vi "Autonomous Independent.vi"() -> ()   [LabVIEW 2012]
doc: "This VI is called when autonomous begins, and will automatically be terminated when autonomous ends. You can carry out timed or sensor driven robot movement independently without needing to return to the caller."
uses:
  <vilib>/Rock Robotics/WPI/Relay/WPI_RelayValue.ctl
  Robot Global Data.vi
  <vilib>/Rock Robotics/WPI/RobotDrive/WPI_RobotDriveGetSetRefNum.vi
  <vilib>/Rock Robotics/WPI/RobotDrive/WPI_RobotDriveArcadeDrive_Standard(NoSaturation).vi
panel:
  out "Current Movement, for debugging":T1 {"Y Joystick Value" scale=1.0..-1.0; "X Joystick Value" scale=-1.0..1.0}
  in  "Array of robot movements":T2(array[cluster]) {"Y Joystick Value" scale=1.0..-1.0; "X Joystick Value" scale=-1.0..1.0}
  # "Be sure to right-click and choose Data Operations>>Make Current Value default if you want to save the array values with the VI"
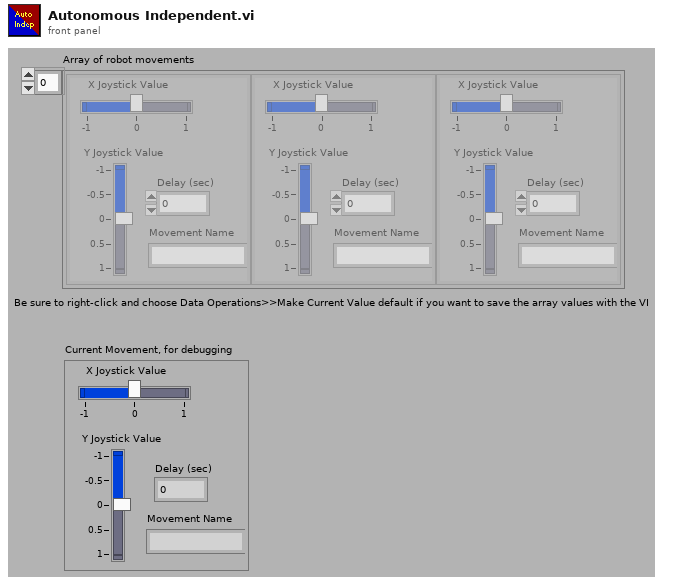
[diagram p1: front panel]
types:
  T1 = cluster{"X Joystick Value":dbl, "Y Joystick Value":dbl, "Delay (sec)":dbl, "Movement Name":string}
  T2 = cluster{"X Joystick Value":dbl, "Y Joystick Value":dbl, "Delay (sec)":dbl, "Movement Name":string}[]
  T3 = typedef "WPI_JoystickDevRef.ctl" = cluster{"Device":T4}
  T4 = typedef "WPI_JoystickDeviceEnum.ctl" = enum16{"USB 1", "USB 2", "USB 3", "USB 4", "Kinect 1", "Kinect 2"}
  T5 = cluster{"axis 1 (x)":dbl, "axis 2 (y)":dbl, "axis 3 (throttle)":dbl, "axis 4":dbl, "axis 5":dbl, "axis 6":dbl}
  T6 = typedef "WPI_RobotDriveDevRef.ctl" = cluster{"DevStatus":errorcluster, "Motors[]":T7[], "Square Inputs":bool, "Max Output":dbl, "Isochronous":bool}
  T7 = typedef "WPI_MotorControlDeviceRef.ctl" = cluster{"DeviceStatus":errorcluster, "Type":enum16{"PWM", "CAN"}, "PWM":cluster{"Digital Module":T8, "PWM Channel":T9, "DeadBand":T10}, "CAN":cluster{"Device Number":u8, "Control Mode":T11, "Semaphore":T12, "Max Vout":dbl}, "Invert":bool, "TransformRef":T13, "InvTransformRef":T13}
  T8 = typedef "FPGA_TypedefDigitalModule.ctl" = enum16{"Digital Module 1", "Digital Module 2"}
  T9 = typedef "FPGA_DIOPWMChannel.ctl" = enum8{"PWM 1", "PWM 2", "PWM 3", "PWM 4", "PWM 5", "PWM 6", "PWM 7", "PWM 8", "PWM 9", "PWM 10", "Invalid"}
  T10 = typedef "WPI_PWMDeadband.ctl" = cluster{"Name":string, "maxPositivePwm":i32, "minPositivePwm":i32, "centerPwm":i32, "maxNegativePwm":i32, "minNegativePwm":i32, "angularRange":u16}
  T11 = typedef "WPI_CANJaguar_ControlMode.ctl" = enum8{"Percent VBus", "Current", "Speed", "Position", "Voltage"}
  T12 = typedef "Semaphore RefNum" = refnum<k1>
  T13 = typedef "WPI_PWMTransform_ConPane.ctl" = refnum<vi>
  T14 = typedef "WPI_RelayValue.ctl" = enum16{"Off", "On", "Forward", "Reverse"}
  T15 = typedef "WPI_RelayDevRef.ctl" = cluster{"DevStatus":errorcluster, "Relay Channel":T16, "Digital Module":T8, "Relay Direction":T17}
  T16 = typedef "FPGA_DIORelayChannel.ctl" = enum8{"Relay 1", "Relay 2", "Relay 3", "Relay 4", "Relay 5", "Relay 6", "Relay 7", "Relay 8", "Invalid"}
  T17 = typedef "WPI_RelayDirection.ctl" = enum16{"Both directions", "Forward only", "Reverse only"}
  T18 = typedef "WPI_EncoderDevRef.ctl" = cluster{"DevStatus":errorcluster, "EncoderIndex":T19, "CounterIndex":T20, "DistancePerCount":dbl, "Decoding Type":T21}
  T19 = typedef "FPGA_EncoderIdx.ctl" = enum8{"Enc 0", "Enc 1", "Enc 2", "Enc 3", "Invalid"}
  T20 = typedef "FPGA_CounterCtrSystemIndex.ctl" = enum8{"Ctr 0", "Ctr 1", "Ctr 2", "Ctr 3", "Ctr 4", "Ctr 5", "Ctr 6", "Ctr 7", "Invalid"}
  T21 = typedef "WPI_EncoderType.ctl" = enum16{"1x", "2x", "4x"}
  T22 = typedef "WPI_ServoDeviceRef.ctl" = cluster{"DeviceStatus":errorcluster, "Digital Module":T8, "PWM Channel":T9, "DeadBand":T10}
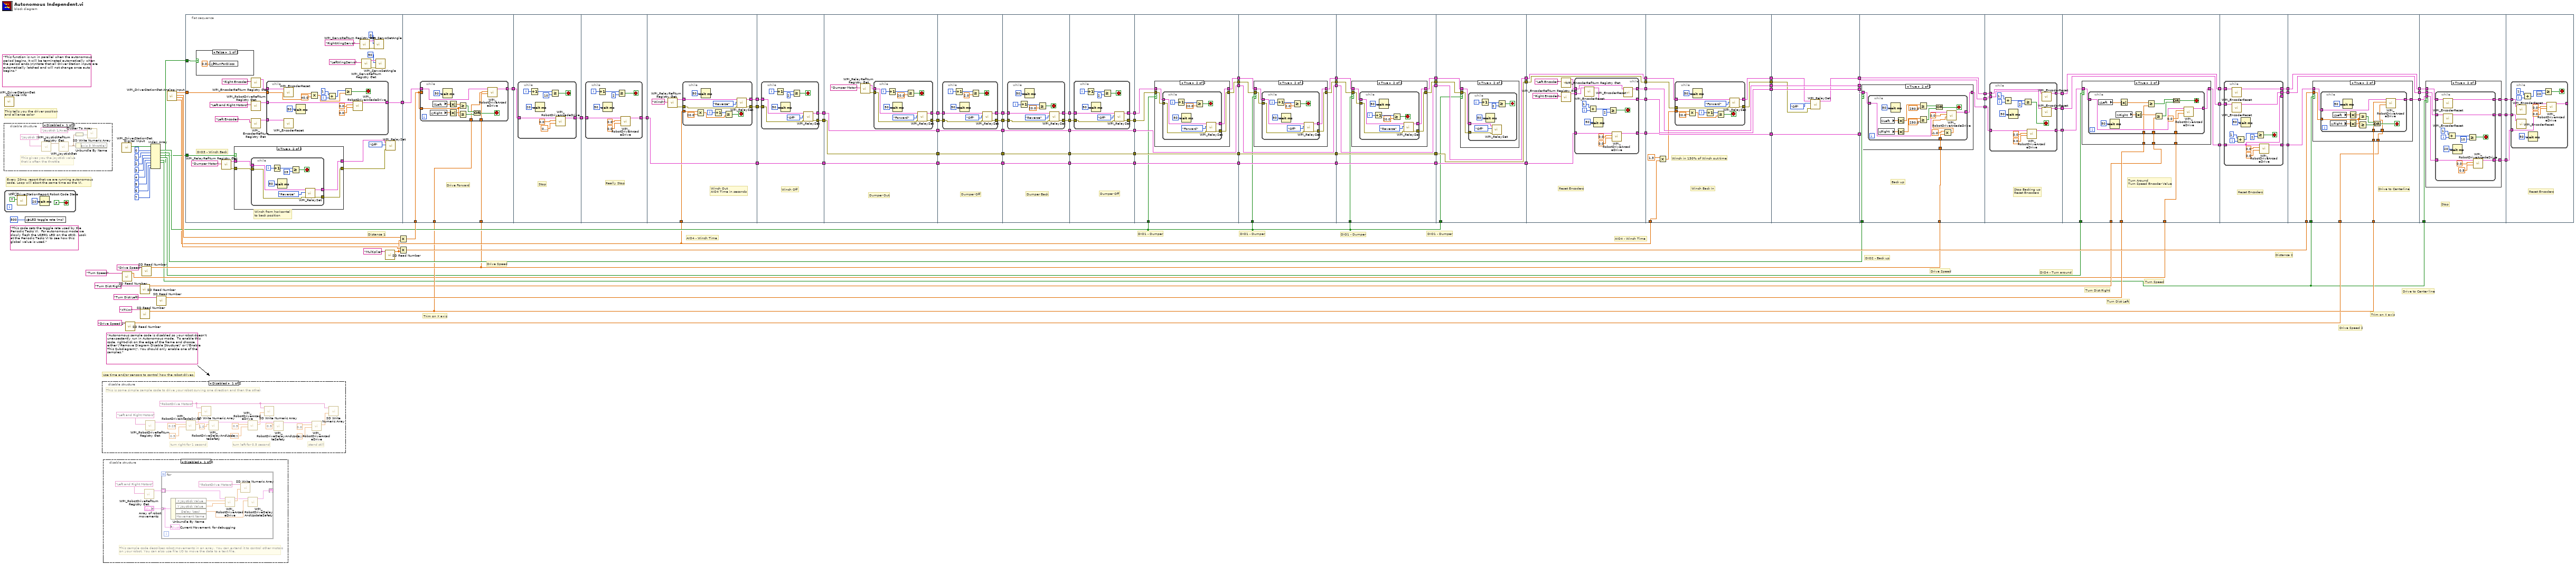
[diagram p0: block diagram]
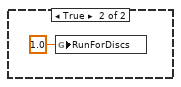
[diagram p3: hidden frame]
diagram:
  (unwired) "This code sets the toggle rate used by the Periodic Tasks VI.  For autonomous mode we slowly flash the USER1 LED on the cRIO.  Look at the Periodic Tasks VI to see how this global value is used."
  (unwired) "Autonomous sample code is disabled so your robot doesn't unexpectantly run in Autonomous mode.  To enable this code, right-click on the edge of the frame and choose either \"Remove Diagram Disable Structure\" or \"Enable This Subdiagram\". You should only enable one of the samples."
  (unwired) "This function is run in parallel when the autonomous period begins. It will be terminated automatically when the period ends.\n\nNote that all Driver Station inputs are automatically latched and will not change once auto begins."
  # "AIO4 - Winch Time"
  # "AIO4 - Winch Time"
  # "Drive to Center line"
  # "DIO4 - Turn around"
  # "DIO2 - Back up"
  # "DIO1 - Dumper"
  # "DIO1 - Dumper"
  # "DIO1 - Dumper"
  # "DIO1 - Dumper"
  # "Trim on X axis"
  # "Drive Speed 2"
  # "Trim on X axis"
  # "Turn Dist Left"
  # "Turn Dist Right"
  # "Turn Speed"
  # "Distance 2"
  # "Distance 1"
  # "Drive Speed"
  # "Drive Speed"
  # "Every 20ms, report that we are running autonomous\ncode. Loop will abort the same time as the VI."
  # "Use time and/or sensors to control how the robot drives."
  # "This tells you the driver position\nand alliance color"
  n1 = disable-structure shown="Disabled" {
    frame Disabled {
      # "This gives you the joystick value\nthat is often the throttle"
      n2 = call <vilib>:"WPI_JoystickRefNum Registry Get.vi"("refnum name"="Joystick 1") -> ("JoystickDevRef"=w120:T3)  [unwired: 1 in, 9 out]
      n3 = call <vilib>:"WPI_JoystickGet.vi"("JoystickDevRef"=w120) -> ("Axes"=w118:T5)  [unwired: 1 in, 5 out]
      n4 = Cluster To Array(cluster=w118) -> (array=w119:dbl[])
      n5 = Unbundle By Name(w118) -> ()  [unwired: 1 out]
      n6 = call <vilib>:"SD Write Numeric Array.vi"("Numeric Array"=w119, "Name"="Joystick 1/Axes") -> ()  [unwired: 8 in, 2 out]
    }
    frame Enabled {
    }
  }
  n7 = call <vilib>:"WPI_DriverStationGet Alliance Info.vi"() -> ()  [unwired: 12 out]
  n8 = while {
    stop <- FALSE stop-if-true
    n9 = call <vilib>:"WPI_DriverStationReport Robot Code State.vi"("Autonomous"=TRUE) -> ()  [unwired: 10 in, 1 out]
    n10 = Wait (ms)(milliseconds to wait=u32 20) -> ()  [unwired: 1 out]
  }
  n11 = global write "Robot Global Data.vi" "LED toggle rate (ms)"(u32 500 ("LED ms toggle rate")) -> ()
  n12 = disable-structure shown="Disabled" {
    frame Disabled {
      w125 = "RobotDrive Motors" ("Name")
      # "This is some simple sample code to drive your robot curving one direction and then the other."
      # "stand still"
      # "turn left for 0.5 second"
      # "turn right for 1 second"
      n13 = call <vilib>:"WPI_RobotDriveRefNum Registry Get.vi"("refnum name"="Left and Right Motors") -> ("RobotDriveDevRef"=w129:T6)  [unwired: 1 in, 9 out]
      n14 = call-poly <vilib>:"WPI_RobotDriveArcadeDrive.vi"("Y axis value"=0.5 ("X axis value"), "X axis value"=0.25, "RobotDriveDevRef"=w129) -> ("Motor Values"=w128:dbl[], "RobotDriveDevRef"=w136:T6)  [unwired: 1 in, 6 out]
      n15 = call <vilib>:"SD Write Numeric Array.vi"("Numeric Array"=w128, "Name"=w125) -> ()  [unwired: 8 in, 2 out]
      n16 = call <vilib>:"WPI_RobotDriveDelayAndUpdateSafety.vi"("Delay (s)"=1.0, "RobotDriveDevRef"=w136) -> ("RobotDriveDevRef 2"=w135:T6)  [unwired: 8 in, 1 out]
      n17 = call-poly <vilib>:"WPI_RobotDriveArcadeDrive.vi"("Y axis value"=0.25 ("X axis value"), "X axis value"=0.5, "RobotDriveDevRef"=w135) -> ("Motor Values"=w127:dbl[], "RobotDriveDevRef"=w134:T6)  [unwired: 1 in, 6 out]
      n18 = call <vilib>:"SD Write Numeric Array.vi"("Numeric Array"=w127, "Name"=w125) -> ()  [unwired: 8 in, 2 out]
      n19 = call <vilib>:"WPI_RobotDriveDelayAndUpdateSafety.vi"("Delay (s)"=0.5, "RobotDriveDevRef"=w134) -> ("RobotDriveDevRef 2"=w133:T6)  [unwired: 8 in, 1 out]
      n20 = call-poly <vilib>:"WPI_RobotDriveArcadeDrive.vi"("Y axis value"=0.0 ("X axis value"), "X axis value"=0.0, "RobotDriveDevRef"=w133) -> ("Motor Values"=w126:dbl[])  [unwired: 1 in, 7 out]
      n21 = call <vilib>:"SD Write Numeric Array.vi"("Numeric Array"=w126, "Name"=w125) -> ()  [unwired: 8 in, 2 out]
    }
    frame Enabled {
    }
  }
  n22 = disable-structure shown="Disabled" {
    frame Disabled {
      # "This sample code describes robot movements in an array. You can extend it to control other motors\non your robot. You can also use file I/O to move the data to a text file."
      n23 = call <vilib>:"WPI_RobotDriveRefNum Registry Get.vi"("refnum name"="Left and Right Motors") -> ("RobotDriveDevRef"=w144:T6)  [unwired: 1 in, 9 out]
      n24 = for {
        shift-right: [w150] -> _
        shift-left: w144 -> [w151]
        tunnel: "Array of robot movements" -> [w146] mode=indexing
        n25 = Unbundle By Name(w146) -> ("X Joystick Value"=w149:dbl, "Y Joystick Value"=w148:dbl, "Delay (sec)"=w147:dbl)  [unwired: 1 out]
        n26 = call-poly <vilib>:"WPI_RobotDriveArcadeDrive.vi"("Y axis value"=w148, "X axis value"=w149, "RobotDriveDevRef"=w151) -> ("Motor Values"=w153:dbl[], "RobotDriveDevRef"=w152:T6)  [unwired: 1 in, 6 out]
        n27 = call <vilib>:"SD Write Numeric Array.vi"("Numeric Array"=w153, "Name"="RobotDrive Motors") -> ()  [unwired: 8 in, 2 out]
        n28 = call <vilib>:"WPI_RobotDriveDelayAndUpdateSafety.vi"("Delay (s)"=w147, "RobotDriveDevRef"=w152) -> ("RobotDriveDevRef 2"=w150:T6)  [unwired: 8 in, 1 out]
        "Current Movement, for debugging" <- w146
      }
    }
    frame Enabled {
    }
  }
  n29 = call <vilib>:"WPI_DriverStationGet Digital Input.vi"() -> ("Driver Station Digital Input (1-8)"=w35:bool[])  [unwired: 11 out]
  n30 = call <vilib>:"SD Read Number.vi"("Name"="Turn Speed") -> ("Numeric"=w6:dbl)  [unwired: 8 in, 2 out]
  n31 = call <vilib>:"SD Read Number.vi"("Name"="Drive Speed 2") -> ("Numeric"=w4:dbl)  [unwired: 8 in, 2 out]
  n32 = call <vilib>:"SD Read Number.vi"("Name"="Turn Dist Right") -> ("Numeric"=w8:dbl)  [unwired: 8 in, 2 out]
  n33 = call <vilib>:"SD Read Number.vi"("Name"="XTrim") -> ("Numeric"=w10:dbl)  [unwired: 8 in, 2 out]
  n34 = call <vilib>:"SD Read Number.vi"("Name"="Drive Speed") -> ("Numeric"=w12:dbl)  [unwired: 8 in, 2 out]
  n35 = Index Array(array=w35, index #1=0 ("index"), index #2=1 ("index"), index #3=2 ("index"), index #4=3 ("index"), index #5=4 ("index"), index #6=5 ("index"), index #7=6 ("index"), index #8=7 ("index")) -> (element #1=w21:bool, element #2=w17:bool, element #3=w16:bool, element #4=w3:bool, element #5=w2:bool, element #6=w1:bool)  [unwired: 2 out]
  n36 = call <vilib>:"SD Read Number.vi"("Name"="Turn Dist Left") -> ("Numeric"=w13:dbl)  [unwired: 8 in, 2 out]
  n37 = call <vilib>:"WPI_DriverStationGet Analog Input.vi"() -> ("Analog 4 (V)"=w15:dbl, "Analog 3 (V)"=w23:dbl, "Analog 2 (V)"=w24:dbl, "Analog 1 (V)"=w25:dbl)  [unwired: 8 out]
  n38 = flat-sequence {
    tunnel: [w173] -> w115
    tunnel: w25 -> [w172]
    tunnel: w16 -> [w171]
    tunnel: w1 -> [w164]
    tunnel: w115 -> [w215]
    tunnel: w26 -> [w213]
    tunnel: [w214] -> w114
    tunnel: w12 -> [w212]
    tunnel: w10 -> [w211]
    tunnel: w114 -> [w230]
    tunnel: [w229] -> w113
    tunnel: w113 -> [w241]
    tunnel: [w240] -> w112
    tunnel: [w254] -> w111
    tunnel: [w253] -> w110
    tunnel: [w252] -> w109
    tunnel: w112 -> [w252]
    tunnel: w15 -> [w251]
    tunnel: w111 -> [w274]
    tunnel: w110 -> [w273]
    tunnel: [w272] -> w108
    tunnel: [w271] -> w107
    tunnel: [w270] -> w106
    tunnel: w109 -> [w270]
    tunnel: w108 -> [w292]
    tunnel: [w292] -> w105
    tunnel: w107 -> [w291]
    tunnel: [w291] -> w104
    tunnel: w106 -> [w290]
    tunnel: [w290] -> w103
    tunnel: [w289] -> w102
    tunnel: [w288] -> w101
    tunnel: [w309] -> w100
    tunnel: [w308] -> w99
    tunnel: [w307] -> w98
    tunnel: w105 -> [w307]
    tunnel: w104 -> [w306]
    tunnel: [w306] -> w97
    tunnel: [w305] -> w96
    tunnel: w103 -> [w305]
    tunnel: w102 -> [w304]
    tunnel: w101 -> [w303]
    tunnel: w100 -> [w326]
    tunnel: w99 -> [w325]
    tunnel: [w324] -> w95
    tunnel: [w323] -> w94
    tunnel: [w322] -> w93
    tunnel: w98 -> [w322]
    tunnel: w97 -> [w321]
    tunnel: [w321] -> w92
    tunnel: [w320] -> w91
    tunnel: w96 -> [w320]
    tunnel: w95 -> [w343]
    tunnel: w94 -> [w342]
    tunnel: [w341] -> w90
    tunnel: w93 -> [w341]
    tunnel: w92 -> [w340]
    tunnel: [w340] -> w89
    tunnel: [w339] -> w88
    tunnel: w91 -> [w339]
    tunnel: [w338] -> w87
    tunnel: [w337] -> w86
    tunnel: w90 -> [w361]
    tunnel: [w361] -> w85
    tunnel: w89 -> [w360]
    tunnel: [w360] -> w84
    tunnel: w88 -> [w359]
    tunnel: [w359] -> w83
    tunnel: w87 -> [w358]
    tunnel: w86 -> [w357]
    tunnel: [w356] -> w82
    tunnel: [w355] -> w81
    tunnel: w21 -> [w354]
    tunnel: w85 -> [w385]
    tunnel: [w385] -> w80
    tunnel: w84 -> [w384]
    tunnel: [w384] -> w79
    tunnel: w83 -> [w383]
    tunnel: [w383] -> w78
    tunnel: w82 -> [w382]
    tunnel: w81 -> [w381]
    tunnel: [w380] -> w77
    tunnel: [w379] -> w76
    tunnel: w21 -> [w378]
    tunnel: w80 -> [w409]
    tunnel: [w409] -> w75
    tunnel: w79 -> [w408]
    tunnel: [w408] -> w74
    tunnel: w78 -> [w407]
    tunnel: [w407] -> w73
    tunnel: w77 -> [w406]
    tunnel: w76 -> [w405]
    tunnel: [w404] -> w72
    tunnel: [w403] -> w71
    tunnel: w21 -> [w402]
    tunnel: w75 -> [w431]
    tunnel: [w431] -> w70
    tunnel: w74 -> [w430]
    tunnel: [w430] -> w69
    tunnel: w73 -> [w429]
    tunnel: [w429] -> w68
    tunnel: w72 -> [w428]
    tunnel: w71 -> [w427]
    tunnel: w21 -> [w426]
    tunnel: w70 -> [w451]
    tunnel: [w451] -> w67
    tunnel: w69 -> [w450]
    tunnel: [w450] -> w66
    tunnel: w68 -> [w449]
    tunnel: [w448] -> w65
    tunnel: [w443] -> w64
    tunnel: [w442] -> w63
    tunnel: w67 -> [w475]
    tunnel: w66 -> [w474]
    tunnel: [w473] -> w62
    tunnel: [w472] -> w61
    tunnel: w65 -> [w469]
    tunnel: [w471] -> w60
    tunnel: w64 -> [w471]
    tunnel: [w470] -> w59
    tunnel: w63 -> [w470]
    tunnel: [w469] -> w58
    tunnel: w15 -> [w467]
    tunnel: w62 -> [w489]
    tunnel: [w488] -> w57
    tunnel: w61 -> [w491]
    tunnel: w60 -> [w494]
    tunnel: [w494] -> w56
    tunnel: w59 -> [w493]
    tunnel: [w493] -> w55
    tunnel: w58 -> [w492]
    tunnel: [w492] -> w54
    tunnel: w57 -> [_]
    tunnel: w56 -> [w500]
    tunnel: [w500] -> w53
    tunnel: w55 -> [w499]
    tunnel: [w499] -> w52
    tunnel: w54 -> [w498]
    tunnel: w17 -> [w497]
    tunnel: [w496] -> w51
    tunnel: w12 -> [w495]
    tunnel: w53 -> [w526]
    tunnel: w52 -> [w525]
    tunnel: [w524] -> w50
    tunnel: [w523] -> w49
    tunnel: [w522] -> w48
    tunnel: w51 -> [w521]
    tunnel: [w545] -> w47
    tunnel: [w544] -> w46
    tunnel: [w548] -> w45
    tunnel: w3 -> [w547]
    tunnel: w50 -> [w546]
    tunnel: w49 -> [w545]
    tunnel: w48 -> [w544]
    tunnel: w13 -> [w543]
    tunnel: w8 -> [w542]
    tunnel: w6 -> [w541]
    tunnel: w47 -> [w574]
    tunnel: w46 -> [w573]
    tunnel: w45 -> [w572]
    tunnel: [w571] -> w44
    tunnel: [w570] -> w43
    tunnel: [w569] -> w42
    tunnel: w44 -> [w596]
    tunnel: [w595] -> w41
    tunnel: w43 -> [w595]
    tunnel: [w594] -> w40
    tunnel: w42 -> [w594]
    tunnel: [w593] -> w39
    tunnel: w22 -> [w592]
    tunnel: w2 -> [w591]
    tunnel: w4 -> [w589]
    tunnel: w10 -> [w590]
    tunnel: w41 -> [w622]
    tunnel: w40 -> [w621]
    tunnel: w39 -> [w620]
    tunnel: [w619] -> w38
    tunnel: [w618] -> w37
    tunnel: [w617] -> w36
    tunnel: w2 -> [w616]
    tunnel: w38 -> [w648]
    tunnel: w37 -> [w647]
    tunnel: w36 -> [w646]
    frame #0 {
      # "DIO3 - Winch Back"
      # "Winch from horizontal\nto back position"
      n39 = case shown="False" w164 {
        frame False {
          n40 = global write "Robot Global Data.vi" "RunForDiscs"(0.0 ("RunForDiscs")) -> ()
        }
        frame True {
          n41 = global write "Robot Global Data.vi" "RunForDiscs"(1.0 ("RunForDiscs")) -> ()
        }
      }
      n42 = call <vilib>:"WPI_RelayRefNum Registry Get.vi"("refnum name"="Dumper Motor") -> ("error out"=w168:errorcluster, "RelayDevRef"=w166:T15)  [unwired: 9 in]
      n43 = case shown="True" w171 {
        tunnel: [w182 w184] -> w169
        tunnel: [w181 w186] -> w165
        tunnel: w168 -> [w182 w185]
        tunnel: w166 -> [w181 w183]
        frame False {
        }
        frame True {
          n44 = while {
            tunnel: w185 -> [w192]
            tunnel: [w189] -> w186
            tunnel: [w188] -> w184
            tunnel: w183 -> [w187]
            i -> [w195]
            stop <- w194 stop-if-true
            n45 = Increment(x=w195) -> (x+1=w191:i32)
            n46 = Wait (ms)(milliseconds to wait=u32 50) -> ()  [unwired: 1 out]
            n47 = Greater Or Equal?(x=w191, y=25 ("x")) -> (x >= y?=w194:bool)
            n48 = call <vilib>:"WPI_RelaySet.vi"("error in (no error)"=w192, "RelayValue"=WPI_RelayValue."Reverse", "RelayDevRef"=w187) -> ("error out"=w188:errorcluster, "RelayDevRef"=w189:T15)  [unwired: 7 in]
          }
        }
      }
      n49 = call <vilib>:"WPI_EncoderRefNum Registry Get.vi"("refnum name"="Right Encoder") -> ("EncoderDevRef"=w175:T18)  [unwired: 9 in, 1 out]
      n50 = call <vilib>:"WPI_RobotDriveRefNum Registry Get.vi"("refnum name"="Left and Right Motors") -> ("RobotDriveDevRef"=w177:T6)  [unwired: 9 in, 1 out]
      n51 = call <vilib>:"WPI_EncoderRefNum Registry Get.vi"("refnum name"="Left Encoder") -> ("EncoderDevRef"=w176:T18)  [unwired: 9 in, 1 out]
      n52 = while {
        tunnel: w177 -> [w204]
        tunnel: w176 -> [w203]
        tunnel: w175 -> [w202]
        tunnel: [w201] -> w173
        tunnel: w172 -> [w198]
        i -> [w207]
        stop <- w205 stop-if-true
        n53 = call <vilib>:"WPI_EncoderReset.vi"("EncoderDevRef"=w202) -> ()  [unwired: 9 in, 2 out]
        n54 = call <vilib>:"WPI_EncoderReset.vi"("EncoderDevRef"=w203) -> ()  [unwired: 9 in, 2 out]
        n55 = Wait (ms)(milliseconds to wait=u32 50) -> ()  [unwired: 1 out]
        n56 = Multiply(x=w198, y=40.0) -> (x*y=w199:dbl)
        n57 = Add(x=1, y=w207) -> (x+y=w200:i32)
        n58 = Greater Or Equal?(x=w200, y=w199) -> (x >= y?=w205:bool)
        n59 = call-poly <vilib>:"WPI_RobotDriveArcadeDrive.vi"("Y axis value"=0.0, "X axis value"=0.0, "RobotDriveDevRef"=w204) -> ("RobotDriveDevRef"=w201:T6)  [unwired: 6 in, 2 out]
      }
      n60 = call <vilib>:"WPI_ServoRefNum Registry Get.vi"("refnum name"="RightWingServo") -> ("error out"=w162:errorcluster, "ServoDeviceRef"=w161:T22)  [unwired: 9 in]
      n61 = call <vilib>:"WPI_ServoRefNum Registry Get.vi"("refnum name"="LeftWingServo") -> ("error out"=w159:errorcluster, "ServoDeviceRef"=w158:T22)  [unwired: 9 in]
      n62 = call <vilib>:"WPI_ServoSetAngle.vi"("error in (no error)"=w162, "Angle"=0, "ServoDeviceRef"=w161) -> ()  [unwired: 7 in, 2 out]
      n63 = call <vilib>:"WPI_ServoSetAngle.vi"("error in (no error)"=w159, "Angle"=90, "ServoDeviceRef"=w158) -> ()  [unwired: 7 in, 2 out]
      n64 = call <vilib>:"WPI_RelaySet.vi"("error in (no error)"=w169, "RelayValue"=WPI_RelayValue."Off", "RelayDevRef"=w165) -> ()  [unwired: 7 in, 2 out]
    }
    frame #1 {
      # "Drive Forward"
      n65 = while {
        tunnel: w215 -> [w227]
        tunnel: w213 -> [w220]
        tunnel: [w226] -> w214
        tunnel: w213 -> [_]
        tunnel: w212 -> [w217]
        tunnel: w211 -> [w216]
        stop <- w221 stop-if-true
        n66 = global read "Robot Global Data.vi" "Right"() -> (w224:dbl)
        n67 = global read "Robot Global Data.vi" "Left"() -> (w225:dbl)
        n68 = Wait (ms)(milliseconds to wait=u32 50) -> ()  [unwired: 1 out]
        n69 = Absolute Value(x=w225) -> (abs(x)=w218:dbl)
        n70 = Absolute Value(x=w224) -> (abs(x)=w219:dbl)
        n71 = Greater Or Equal?(x=w218, y=w220) -> (x >= y?=w223:bool)
        n72 = Greater Or Equal?(x=w219, y=w220) -> (x >= y?=w222:bool)
        n73 = Or(x=w223, y=w222) -> (x .or. y?=w221:bool)
        n74 = call-poly <vilib>:"WPI_RobotDriveArcadeDrive.vi"("Y axis value"=w217, "X axis value"=w216, "RobotDriveDevRef"=w227) -> ("RobotDriveDevRef"=w226:T6)  [unwired: 6 in, 2 out]
      }
    }
    frame #2 {
      # "Stop"
      n75 = while {
        tunnel: w230 -> [w237]
        tunnel: [w231] -> w229
        i -> [w235]
        stop <- w232 stop-if-true
        n76 = Increment(x=w235) -> (x+1=w234:i32)
        n77 = Wait (ms)(milliseconds to wait=u32 20) -> ()  [unwired: 1 out]
        n78 = Greater Or Equal?(x=w234, y=10) -> (x >= y?=w232:bool)
        n79 = call-poly <vilib>:"WPI_RobotDriveArcadeDrive.vi"("Y axis value"=0.30000000000000004, "X axis value"=0.0, "RobotDriveDevRef"=w237) -> ("RobotDriveDevRef"=w231:T6)  [unwired: 6 in, 2 out]
      }
    }
    frame #3 {
      # "Really Stop"
      n80 = while {
        tunnel: w241 -> [w248]
        tunnel: [w242] -> w240
        i -> [w246]
        stop <- w243 stop-if-true
        n81 = Increment(x=w246) -> (x+1=w245:i32)
        n82 = Wait (ms)(milliseconds to wait=u32 50) -> ()  [unwired: 1 out]
        n83 = Greater Or Equal?(x=w245, y=2) -> (x >= y?=w243:bool)
        n84 = call-poly <vilib>:"WPI_RobotDriveArcadeDrive.vi"("Y axis value"=0.0, "X axis value"=0.0, "RobotDriveDevRef"=w248) -> ("RobotDriveDevRef"=w242:T6)  [unwired: 6 in, 2 out]
      }
    }
    frame #4 {
      # "Winch Out\nAIO4 Time in seconds"
      n85 = call <vilib>:"WPI_RelayRefNum Registry Get.vi"("refnum name"="Winch") -> ("error out"=w255:errorcluster, "RelayDevRef"=w256:T15)  [unwired: 9 in]
      n86 = while {
        tunnel: w256 -> [w265]
        tunnel: w255 -> [w264]
        tunnel: [w262] -> w254
        tunnel: [w261] -> w253
        tunnel: w251 -> [w260]
        i -> [w268]
        stop <- w267 stop-if-true
        n87 = Multiply(x=w260, y=20.0) -> (x*y=w258:dbl)
        n88 = Wait (ms)(milliseconds to wait=u32 50) -> ()  [unwired: 1 out]
        n89 = Increment(x=w268) -> (x+1=w263:i32)
        n90 = Greater Or Equal?(x=w263, y=w258) -> (x >= y?=w267:bool)
        n91 = call <vilib>:"WPI_RelaySet.vi"("error in (no error)"=w264, "RelayValue"=WPI_RelayValue."Reverse", "RelayDevRef"=w265) -> ("error out"=w261:errorcluster, "RelayDevRef"=w262:T15)  [unwired: 7 in]
      }
    }
    frame #5 {
      # "Winch Off"
      n92 = while {
        tunnel: w274 -> [w278]
        tunnel: w273 -> [w277]
        tunnel: [w276] -> w272
        tunnel: [w275] -> w271
        i -> [w283]
        stop <- w282 stop-if-true
        n93 = Increment(x=w283) -> (x+1=w280:i32)
        n94 = Wait (ms)(milliseconds to wait=u32 50) -> ()  [unwired: 1 out]
        n95 = Greater Or Equal?(x=w280, y=2 ("x")) -> (x >= y?=w282:bool)
        n96 = call <vilib>:"WPI_RelaySet.vi"("error in (no error)"=w277, "RelayValue"=WPI_RelayValue."Off", "RelayDevRef"=w278) -> ("error out"=w275:errorcluster, "RelayDevRef"=w276:T15)  [unwired: 7 in]
      }
    }
    frame #6 {
      # "Dumper Out"
      n97 = call <vilib>:"WPI_RelayRefNum Registry Get.vi"("refnum name"="Dumper Motor") -> ("error out"=w285:errorcluster, "RelayDevRef"=w286:T15)  [unwired: 9 in]
      n98 = while {
        tunnel: [w296] -> w289
        tunnel: [w295] -> w288
        tunnel: w286 -> [w294]
        tunnel: w285 -> [w293]
        i -> [w300]
        stop <- w299 stop-if-true
        n99 = Increment(x=w300) -> (x+1=w298:i32)
        n100 = Wait (ms)(milliseconds to wait=u32 50) -> ()  [unwired: 1 out]
        n101 = Greater Or Equal?(x=w298, y=20.0 ("x")) -> (x >= y?=w299:bool)
        n102 = call <vilib>:"WPI_RelaySet.vi"("error in (no error)"=w293, "RelayValue"=WPI_RelayValue."Forward", "RelayDevRef"=w294) -> ("error out"=w295:errorcluster, "RelayDevRef"=w296:T15)  [unwired: 7 in]
      }
    }
    frame #7 {
      # "Dumper Off"
      n103 = while {
        tunnel: [w313] -> w309
        tunnel: [w312] -> w308
        tunnel: w304 -> [w311]
        tunnel: w303 -> [w310]
        i -> [w316]
        stop <- w317 stop-if-true
        n104 = Increment(x=w316) -> (x+1=w314:i32)
        n105 = Wait (ms)(milliseconds to wait=u32 50) -> ()  [unwired: 1 out]
        n106 = Greater Or Equal?(x=w314, y=2.0 ("x")) -> (x >= y?=w317:bool)
        n107 = call <vilib>:"WPI_RelaySet.vi"("error in (no error)"=w310, "RelayValue"=WPI_RelayValue."Off", "RelayDevRef"=w311) -> ("error out"=w312:errorcluster, "RelayDevRef"=w313:T15)  [unwired: 7 in]
      }
    }
    frame #8 {
      # "Dumper Back"
      n108 = while {
        tunnel: w326 -> [w330]
        tunnel: w325 -> [w329]
        tunnel: [w328] -> w324
        tunnel: [w327] -> w323
        i -> [w333]
        stop <- w334 stop-if-true
        n109 = Increment(x=w333) -> (x+1=w331:i32)
        n110 = Wait (ms)(milliseconds to wait=u32 50) -> ()  [unwired: 1 out]
        n111 = Greater Or Equal?(x=w331, y=20.0 ("x")) -> (x >= y?=w334:bool)
        n112 = call <vilib>:"WPI_RelaySet.vi"("error in (no error)"=w329, "RelayValue"=WPI_RelayValue."Reverse", "RelayDevRef"=w330) -> ("error out"=w327:errorcluster, "RelayDevRef"=w328:T15)  [unwired: 7 in]
      }
    }
    frame #9 {
      # "Dumper Off"
      n113 = while {
        tunnel: w343 -> [w347]
        tunnel: w342 -> [w346]
        tunnel: [w345] -> w338
        tunnel: [w344] -> w337
        i -> [w352]
        stop <- w351 stop-if-true
        n114 = Increment(x=w352) -> (x+1=w349:i32)
        n115 = Wait (ms)(milliseconds to wait=u32 50) -> ()  [unwired: 1 out]
        n116 = Greater Or Equal?(x=w349, y=2 ("x")) -> (x >= y?=w351:bool)
        n117 = call <vilib>:"WPI_RelaySet.vi"("error in (no error)"=w346, "RelayValue"=WPI_RelayValue."Off", "RelayDevRef"=w347) -> ("error out"=w344:errorcluster, "RelayDevRef"=w345:T15)  [unwired: 7 in]
      }
    }
    frame #10 {
      n118 = case shown="True" w354 {
        tunnel: w358 -> [w363 w367]
        tunnel: w357 -> [w362 w366]
        tunnel: [w363 w365] -> w356
        tunnel: [w362 w364] -> w355
        frame False {
        }
        frame True {
          n119 = while {
            tunnel: [w371] -> w365
            tunnel: [w370] -> w364
            tunnel: w367 -> [w369]
            tunnel: w366 -> [w368]
            i -> [w375]
            stop <- w374 stop-if-true
            n120 = Increment(x=w375) -> (x+1=w373:i32)
            n121 = Wait (ms)(milliseconds to wait=u32 50) -> ()  [unwired: 1 out]
            n122 = Greater Or Equal?(x=w373, y=20.0 ("x")) -> (x >= y?=w374:bool)
            n123 = call <vilib>:"WPI_RelaySet.vi"("error in (no error)"=w368, "RelayValue"=WPI_RelayValue."Forward", "RelayDevRef"=w369) -> ("error out"=w370:errorcluster, "RelayDevRef"=w371:T15)  [unwired: 7 in]
          }
        }
      }
    }
    frame #11 {
      n124 = case shown="True" w378 {
        tunnel: w382 -> [w387 w391]
        tunnel: w381 -> [w386 w390]
        tunnel: [w387 w389] -> w380
        tunnel: [w386 w388] -> w379
        frame False {
        }
        frame True {
          n125 = while {
            tunnel: [w395] -> w389
            tunnel: [w394] -> w388
            tunnel: w391 -> [w393]
            tunnel: w390 -> [w392]
            i -> [w398]
            stop <- w399 stop-if-true
            n126 = Increment(x=w398) -> (x+1=w396:i32)
            n127 = Wait (ms)(milliseconds to wait=u32 50) -> ()  [unwired: 1 out]
            n128 = Greater Or Equal?(x=w396, y=2.0 ("x")) -> (x >= y?=w399:bool)
            n129 = call <vilib>:"WPI_RelaySet.vi"("error in (no error)"=w392, "RelayValue"=WPI_RelayValue."Off", "RelayDevRef"=w393) -> ("error out"=w394:errorcluster, "RelayDevRef"=w395:T15)  [unwired: 7 in]
          }
        }
      }
    }
    frame #12 {
      n130 = case shown="True" w402 {
        tunnel: w406 -> [w411 w415]
        tunnel: w405 -> [w410 w414]
        tunnel: [w411 w413] -> w404
        tunnel: [w410 w412] -> w403
        frame False {
        }
        frame True {
          n131 = while {
            tunnel: [w419] -> w413
            tunnel: [w418] -> w412
            tunnel: w415 -> [w417]
            tunnel: w414 -> [w416]
            i -> [w422]
            stop <- w423 stop-if-true
            n132 = Increment(x=w422) -> (x+1=w420:i32)
            n133 = Wait (ms)(milliseconds to wait=u32 50) -> ()  [unwired: 1 out]
            n134 = Greater Or Equal?(x=w420, y=20.0 ("x")) -> (x >= y?=w423:bool)
            n135 = call <vilib>:"WPI_RelaySet.vi"("error in (no error)"=w416, "RelayValue"=WPI_RelayValue."Reverse", "RelayDevRef"=w417) -> ("error out"=w418:errorcluster, "RelayDevRef"=w419:T15)  [unwired: 7 in]
          }
        }
      }
    }
    frame #13 {
      n136 = case shown="True" w426 {
        tunnel: w428 -> [_ w433]
        tunnel: w427 -> [_ w432]
        frame False {
        }
        frame True {
          n137 = while {
            tunnel: w433 -> [w435]
            tunnel: w432 -> [w434]
            i -> [w440]
            stop <- w439 stop-if-true
            n138 = Increment(x=w440) -> (x+1=w437:i32)
            n139 = Wait (ms)(milliseconds to wait=u32 50) -> ()  [unwired: 1 out]
            n140 = call <vilib>:"WPI_RelaySet.vi"("error in (no error)"=w434, "RelayValue"=WPI_RelayValue."Off", "RelayDevRef"=w435) -> ()  [unwired: 7 in, 2 out]
            n141 = Greater Or Equal?(x=w437, y=2 ("x")) -> (x >= y?=w439:bool)
          }
        }
      }
    }
    frame #14 {
      # "Reset Encoders"
      n142 = call <vilib>:"WPI_EncoderRefNum Registry Get.vi"("refnum name"="Left Encoder") -> ("EncoderDevRef"=w445:T18)  [unwired: 9 in, 1 out]
      n143 = call <vilib>:"WPI_EncoderRefNum Registry Get.vi"("refnum name"="Right Encoder") -> ("EncoderDevRef"=w444:T18)  [unwired: 9 in, 1 out]
      n144 = while {
        tunnel: [w457] -> w443
        tunnel: [w456] -> w442
        tunnel: w449 -> [w455]
        tunnel: [w454] -> w448
        tunnel: w445 -> [w453]
        tunnel: w444 -> [w452]
        i -> [w462]
        stop <- w460 stop-if-true
        n145 = call <vilib>:"WPI_EncoderReset.vi"("EncoderDevRef"=w452) -> ("EncoderDevRef"=w456:T18)  [unwired: 9 in, 1 out]
        n146 = Add(x=1, y=w462) -> (x+y=w459:i32)
        n147 = Wait (ms)(milliseconds to wait=u32 50) -> ()  [unwired: 1 out]
        n148 = Greater Or Equal?(x=w459, y=2 ("x")) -> (x >= y?=w460:bool)
        n149 = call-poly <vilib>:"WPI_RobotDriveArcadeDrive.vi"("Y axis value"=0.0, "X axis value"=0.0, "RobotDriveDevRef"=w455) -> ("RobotDriveDevRef"=w454:T6)  [unwired: 6 in, 2 out]
        n150 = call <vilib>:"WPI_EncoderReset.vi"("EncoderDevRef"=w453) -> ("EncoderDevRef"=w457:T18)  [unwired: 9 in, 1 out]
      }
    }
    frame #15 {
      # "Winch in 130% of Winch out time"
      # "Winch Back In"
      n151 = Multiply(x=1.3, y=w467) -> (x*y=w466:dbl)
      n152 = while {
        tunnel: w475 -> [w482]
        tunnel: w474 -> [w481]
        tunnel: [w480] -> w473
        tunnel: [w479] -> w472
        tunnel: w466 -> [w477]
        i -> [w486]
        stop <- w485 stop-if-true
        n153 = Multiply(x=w477, y=20.0) -> (x*y=w476:dbl)
        n154 = Wait (ms)(milliseconds to wait=u32 50) -> ()  [unwired: 1 out]
        n155 = Increment(x=w486) -> (x+1=w483:i32)
        n156 = Greater Or Equal?(x=w483, y=w476) -> (x >= y?=w485:bool)
        n157 = call <vilib>:"WPI_RelaySet.vi"("error in (no error)"=w481, "RelayValue"=WPI_RelayValue."Forward", "RelayDevRef"=w482) -> ("error out"=w479:errorcluster, "RelayDevRef"=w480:T15)  [unwired: 7 in]
      }
    }
    frame #16 {
      n158 = call <vilib>:"WPI_RelaySet.vi"("error in (no error)"=w491, "RelayValue"=WPI_RelayValue."Off", "RelayDevRef"=w489) -> ("RelayDevRef"=w488:T15)  [unwired: 7 in, 1 out]
    }
    frame #17 {
      # "Back up"
      n159 = case shown="True" w497 {
        tunnel: [w501 w504] -> w496
        tunnel: w498 -> [w501 w503]
        tunnel: w495 -> [_ w502]
        frame False {
        }
        frame True {
          n160 = while {
            tunnel: [w518] -> w504
            tunnel: w503 -> [w508]
            tunnel: w502 -> [w507]
            stop <- w511 stop-if-true
            n161 = global read "Robot Global Data.vi" "Right"() -> (w516:dbl)
            n162 = global read "Robot Global Data.vi" "Left"() -> (w517:dbl)
            n163 = Wait (ms)(milliseconds to wait=u32 50) -> ()  [unwired: 1 out]
            n164 = Absolute Value(x=w517) -> (abs(x)=w515:dbl)
            n165 = Absolute Value(x=w516) -> (abs(x)=w514:dbl)
            n166 = Greater Or Equal?(x=w515, y=250.0) -> (x >= y?=w513:bool)
            n167 = Greater Or Equal?(x=w514, y=250.0) -> (x >= y?=w512:bool)
            n168 = Or(x=w513, y=w512) -> (x .or. y?=w511:bool)
            n169 = Multiply(x=-1.0, y=w507) -> (x*y=w505:dbl)
            n170 = call-poly <vilib>:"WPI_RobotDriveArcadeDrive.vi"("Y axis value"=w505, "X axis value"=0.0, "RobotDriveDevRef"=w508) -> ("RobotDriveDevRef"=w518:T6)  [unwired: 6 in, 2 out]
          }
        }
      }
    }
    frame #18 {
      # "Stop Backing up\nReset Encoders"
      n171 = while {
        tunnel: [w534] -> w524
        tunnel: [w531] -> w522
        tunnel: [w530] -> w523
        tunnel: w526 -> [w529]
        tunnel: w525 -> [w528]
        tunnel: w521 -> [w527]
        i -> [w537]
        stop <- w535 stop-if-true
        n172 = Add(x=1, y=w537) -> (x+y=w533:i32)
        n173 = Wait (ms)(milliseconds to wait=u32 50) -> ()  [unwired: 1 out]
        n174 = Greater Or Equal?(x=w533, y=2 ("x")) -> (x >= y?=w535:bool)
        n175 = call-poly <vilib>:"WPI_RobotDriveArcadeDrive.vi"("Y axis value"=0.0, "X axis value"=0.0, "RobotDriveDevRef"=w527) -> ("RobotDriveDevRef"=w534:T6)  [unwired: 6 in, 2 out]
        n176 = call <vilib>:"WPI_EncoderReset.vi"("EncoderDevRef"=w529) -> ("EncoderDevRef"=w530:T18)  [unwired: 9 in, 1 out]
        n177 = call <vilib>:"WPI_EncoderReset.vi"("EncoderDevRef"=w528) -> ("EncoderDevRef"=w531:T18)  [unwired: 9 in, 1 out]
      }
    }
    frame #19 {
      # "Turn Around\nTurn Speed Encoder Value"
      n178 = case shown="True" w547 {
        tunnel: w546 -> [w549 w554]
        tunnel: [w549 w553] -> w548
        tunnel: w543 -> [_ w552]
        tunnel: w542 -> [_ w551]
        tunnel: w541 -> [_ w550]
        frame False {
        }
        frame True {
          n179 = while {
            tunnel: [w567] -> w553
            tunnel: w554 -> [w558]
            tunnel: w552 -> [w557]
            tunnel: w551 -> [w556]
            tunnel: w550 -> [w555]
            stop <- w560 stop-if-true
            n180 = global read "Robot Global Data.vi" "Left"() -> (w566:dbl)
            n181 = Wait (ms)(milliseconds to wait=u32 50) -> ()  [unwired: 1 out]
            n182 = global read "Robot Global Data.vi" "Right"() -> (w565:dbl)
            n183 = Absolute Value(x=w566) -> (abs(x)=w564:dbl)
            n184 = Absolute Value(x=w565) -> (abs(x)=w563:dbl)
            n185 = Greater Or Equal?(x=w564, y=w557) -> (x >= y?=w562:bool)
            n186 = Greater Or Equal?(x=w563, y=w556) -> (x >= y?=w561:bool)
            n187 = Or(x=w562, y=w561) -> (x .or. y?=w560:bool)
            n188 = call-poly <vilib>:"WPI_RobotDriveArcadeDrive.vi"("Y axis value"=0.0, "X axis value"=w555, "RobotDriveDevRef"=w558) -> ("RobotDriveDevRef"=w567:T6)  [unwired: 6 in, 2 out]
          }
        }
      }
    }
    frame #20 {
      # "Reset Encoders"
      n189 = while {
        tunnel: [w582] -> w571
        tunnel: [w577] -> _
        tunnel: w573 -> [w579]
        tunnel: w574 -> [w578]
        tunnel: w572 -> [w577]
        tunnel: [w576] -> w570
        tunnel: [w575] -> w569
        i -> [w585]
        stop <- w583 stop-if-true
        n190 = call <vilib>:"WPI_EncoderReset.vi"("EncoderDevRef"=w578) -> ("EncoderDevRef"=w576:T18)  [unwired: 9 in, 1 out]
        n191 = call <vilib>:"WPI_EncoderReset.vi"("EncoderDevRef"=w579) -> ("EncoderDevRef"=w575:T18)  [unwired: 9 in, 1 out]
        n192 = Add(x=1, y=w585) -> (x+y=w581:i32)
        n193 = Wait (ms)(milliseconds to wait=u32 50) -> ()  [unwired: 1 out]
        n194 = Greater Or Equal?(x=w581, y=2 ("x")) -> (x >= y?=w583:bool)
        n195 = call-poly <vilib>:"WPI_RobotDriveArcadeDrive.vi"("Y axis value"=0.0, "X axis value"=0.0, "RobotDriveDevRef"=w577) -> ("RobotDriveDevRef"=w582:T6)  [unwired: 6 in, 2 out]
      }
    }
    frame #21 {
      # "Drive to Centerline"
      n196 = case shown="True" w591 {
        tunnel: w596 -> [w597 w602]
        tunnel: [w597 w601] -> w593
        tunnel: w592 -> [_ w600]
        tunnel: w589 -> [_ w598]
        tunnel: w590 -> [_ w599]
        frame False {
        }
        frame True {
          n197 = while {
            tunnel: [w614] -> w601
            tunnel: w602 -> [w606]
            tunnel: w600 -> [w605]
            tunnel: w599 -> [w604]
            tunnel: w598 -> [w603]
            stop <- w607 stop-if-true
            n198 = global read "Robot Global Data.vi" "Right"() -> (w612:dbl)
            n199 = global read "Robot Global Data.vi" "Left"() -> (w613:dbl)
            n200 = Wait (ms)(milliseconds to wait=u32 50) -> ()  [unwired: 1 out]
            n201 = Absolute Value(x=w613) -> (abs(x)=w611:dbl)
            n202 = Absolute Value(x=w612) -> (abs(x)=w610:dbl)
            n203 = Greater Or Equal?(x=w611, y=w605) -> (x >= y?=w609:bool)
            n204 = Greater Or Equal?(x=w610, y=w605) -> (x >= y?=w608:bool)
            n205 = Or(x=w609, y=w608) -> (x .or. y?=w607:bool)
            n206 = call-poly <vilib>:"WPI_RobotDriveArcadeDrive.vi"("Y axis value"=w603, "X axis value"=w604, "RobotDriveDevRef"=w606) -> ("RobotDriveDevRef"=w614:T6)  [unwired: 6 in, 2 out]
          }
        }
      }
    }
    frame #22 {
      # "Stop"
      n207 = case shown="True" w616 {
        tunnel: w622 -> [w625 w631]
        tunnel: w621 -> [w624 w630]
        tunnel: w620 -> [w623 w629]
        tunnel: [w623 w628] -> w619
        tunnel: [w624 w627] -> w618
        tunnel: [w625 w626] -> w617
        frame False {
        }
        frame True {
          n208 = while {
            tunnel: [w639] -> w628
            tunnel: w630 -> [w636]
            tunnel: w631 -> [w635]
            tunnel: w629 -> [w634]
            tunnel: [w633] -> w627
            tunnel: [w632] -> w626
            i -> [w642]
            stop <- w640 stop-if-true
            n209 = call <vilib>:"WPI_EncoderReset.vi"("EncoderDevRef"=w635) -> ("EncoderDevRef"=w632:T18)  [unwired: 9 in, 1 out]
            n210 = call <vilib>:"WPI_EncoderReset.vi"("EncoderDevRef"=w636) -> ("EncoderDevRef"=w633:T18)  [unwired: 9 in, 1 out]
            n211 = Add(x=1, y=w642) -> (x+y=w638:i32)
            n212 = Wait (ms)(milliseconds to wait=u32 20) -> ()  [unwired: 1 out]
            n213 = Greater Or Equal?(x=w638, y=10 ("x")) -> (x >= y?=w640:bool)
            n214 = call-poly <vilib>:"WPI_RobotDriveArcadeDrive.vi"("Y axis value"=0.5, "X axis value"=0.0, "RobotDriveDevRef"=w634) -> ("RobotDriveDevRef"=w639:T6)  [unwired: 6 in, 2 out]
          }
        }
      }
    }
    frame #23 {
      # "Reset Encoders"
      n215 = while {
        tunnel: [w654] -> _
        tunnel: w647 -> [w651]
        tunnel: w646 -> [w650]
        tunnel: w648 -> [w649]
        i -> [w657]
        stop <- w655 stop-if-true
        n216 = call <vilib>:"WPI_EncoderReset.vi"("EncoderDevRef"=w650) -> ()  [unwired: 9 in, 2 out]
        n217 = call <vilib>:"WPI_EncoderReset.vi"("EncoderDevRef"=w651) -> ()  [unwired: 9 in, 2 out]
        n218 = Add(x=1, y=w657) -> (x+y=w653:i32)
        n219 = Wait (ms)(milliseconds to wait=u32 50) -> ()  [unwired: 1 out]
        n220 = Greater Or Equal?(x=w653, y=20 ("x")) -> (x >= y?=w655:bool)
        n221 = call-poly <vilib>:"WPI_RobotDriveArcadeDrive.vi"("Y axis value"=0.0, "X axis value"=0.0, "RobotDriveDevRef"=w649) -> ("RobotDriveDevRef"=w654:T6)  [unwired: 6 in, 2 out]
      }
    }
  }
  n222 = call <vilib>:"SD Read Number.vi"("Name"="Multiplier") -> ("Numeric"=w18:dbl)  [unwired: 8 in, 2 out]
  n223 = Multiply(x=w24, y=w18) -> (x*y=w26:dbl)
  n224 = Multiply(x=w23, y=w18) -> (x*y=w22:dbl)
